vi "02 HEWH MINI Heat Up SM1.vi"(0 "Equipment":T6={"COM Port"="COM3", "MW100"="MW100", "AG34970"="A-34972A", "Chamber"="WT500"}, 2 "Semiphore":T3, 5 "Degree Setting":dbl=58.0, 7 "Flow rate setting":dbl=3.0, 11 "Error In":errorcluster) -> (15 "Error Out":errorcluster)   [LabVIEW 2009]
uses:
  EquipReferences.ctl
  HEWH Tank Indicator.ctl
  PowerElements.ctl
  TestedFlowratesScenarios.ctl
  <vilib>/Platform/fileVersionInfo.llb/FileVersionInformation.ctl
  ValveBankPositions.ctl
  Intellifaucet/Intellfaucet Mode.ctl
  <vilib>/Utility/file.llb/Write To Spreadsheet File (string).vi
  <vilib>/Analysis/NI_AALBase.lvlib
panel:
  in  "Expansion Tank?":bool
  out "FileVersionInfo Out":T1
  in  "Test Condition":T2=enum."Global, Tank"
  out "Chanel List":string
  out "Label Array":string[](array[string])
  out "Use Agilent?":bool
  out "Voltage":dbl=240.0
  out "T4":i32=10000
  out "COM Port":refnum<visa-resource-name>
  out "Serial Data In":string
  out "Error Serial":errorcluster
  in  "StopSerial":bool
  out "LAN IP Address":string="192.168.25.3"
  out "Computer Name":string
  out "Ver.":string
  out "MINI-HEATUP TEST STATUS":string
  in  "Stop":bool
  in  "Help":bool
  out "POWER":T4
  out "Tank Display":T5 {"TC6" format="%.2g"; "TIN" format="%.2g"; "TOUT" format="%.2g"; "Mean" format="%.2f"; "Std Dev" format="%.2f"; "TC5" format="%.2g"; "TC4" format="%.2g"; "TC3" format="%.2g"; "TC2" format="%.2g"; "TC1" format="%.2g"}
  in  "Function Tab":enum32{"Setup", "Test Status", "Charts"}(tab)
  out "MW100":refnum<visa-resource-name>
  out "FileName":path
  in  "Working File Directory":path=path "c:/data"
  out "T1":u32=250
  out "T2":u32=500
  out "T3":u32=500
  in  "Stability Sample Delay(s)":u32=30
  in  "Cold Water Available?":bool=TRUE
  in  "Save File Directory":path=path "c:/data"
  out "Init Complete":bool
  in  "Gallon Limit":dbl=40.0
  in  "Mean Tank Min":dbl=75.0
  in  "Min Tout":dbl=100.0
  in  "GEA2 HyperData":bool
  out "Data Array":string[][](array[string])
  in  "Status Tab":T7(tab)
  out "Flowrate adj":dbl=3.0
  out "Error Out 1":errorcluster
  out "Downspout Flow Chart":dbl(graph)=3.8899999999999997
  out "Temp Band(+/- F)":dbl=50.0
  out "Temp adj":dbl=3.0
  out "Error 5":errorcluster
  out "Downspout Flow Chart":dbl(graph)=3.8899999999999997
  out "Downspout Flow":dbl=3.8899999999999997
  out "Total Flow Out":dbl
  out "5.Top Source Indicator":bool
  in  "Flow Adjust Time (3s)":dbl=1.5
  in  "K(0.1)":dbl=0.1
  out "Gallon Limit 2":dbl=40.0
  out "Mean Tank Min 2":dbl
  out "Min Tout 2":dbl
  out "Heat Source Indicator":bool
  in  "SkipStabilize":bool
  out "error stabilize":errorcluster
  out "Elapsed Time (secs)":dbl format="%.2f"
  out "LoggingStopped":bool=TRUE
  out "Error History":string[](array[string])
  out "Com History":string[](array[string])
  out "error datalogging":errorcluster={"status"=TRUE, "code"=-1073807346, "source"="VISA Read in Gather Test Data.vi"}
  out "St.Logging":bool
  out "Number of Records":i32
  out "Test Data":string[][](array[string])
  in  "Graph Tab":enum32{"Temperature", "Power", "Gallons"}(tab)
  out "Temps":T8(graph) caption="Waveform Chart"
  out "Ave Temp":dbl format="%0.2f"
  out "Watt Chart":T9(graph)
  out "Watts":dbl
  out "Gallons Chart":dbl(graph)
  out "Gallons":dbl
  out "Elapsed Time":dbl format="%<%H:%M:%S>t"
  in  "Stop Logging":bool
  out "Local?":bool
  # "Draw Until:"
  # "Total Gallons Drawn >"
  # "OR"
  # "Mean Temp >="
  # "OR"
  # "Tout <="
  # "\"1.\tAfter unit has been stable for 30+/-5 minutes, Open valve,\n and draw 10.75 +/- .25 gallons of water at a rate of 3+/-.25 gpm.\""
  # "First, Allow the water temp and flow to stabilize in the downspout,\nthen switch to the tank."
  # "\"5.\tOpen valve and draw water at 3+/-.25 gpm until the Upper Element \nenergizes.  Water draw must stop within 5 seconds after Upper Element \nenergizes.  NOTE: when running the unit in e-Heat mode, (no upper \nelement) draw 40+/-0.25 gallons of water.\""
  # "Wait for stabilization.  Checks heat sources every second.  \nIf the heat sources are both off, the water heater is stabilized. \nFor StdElect. Looks at the heating element.  For other heating\nmodes, looks at the RS232 feedback on fans and compressor."
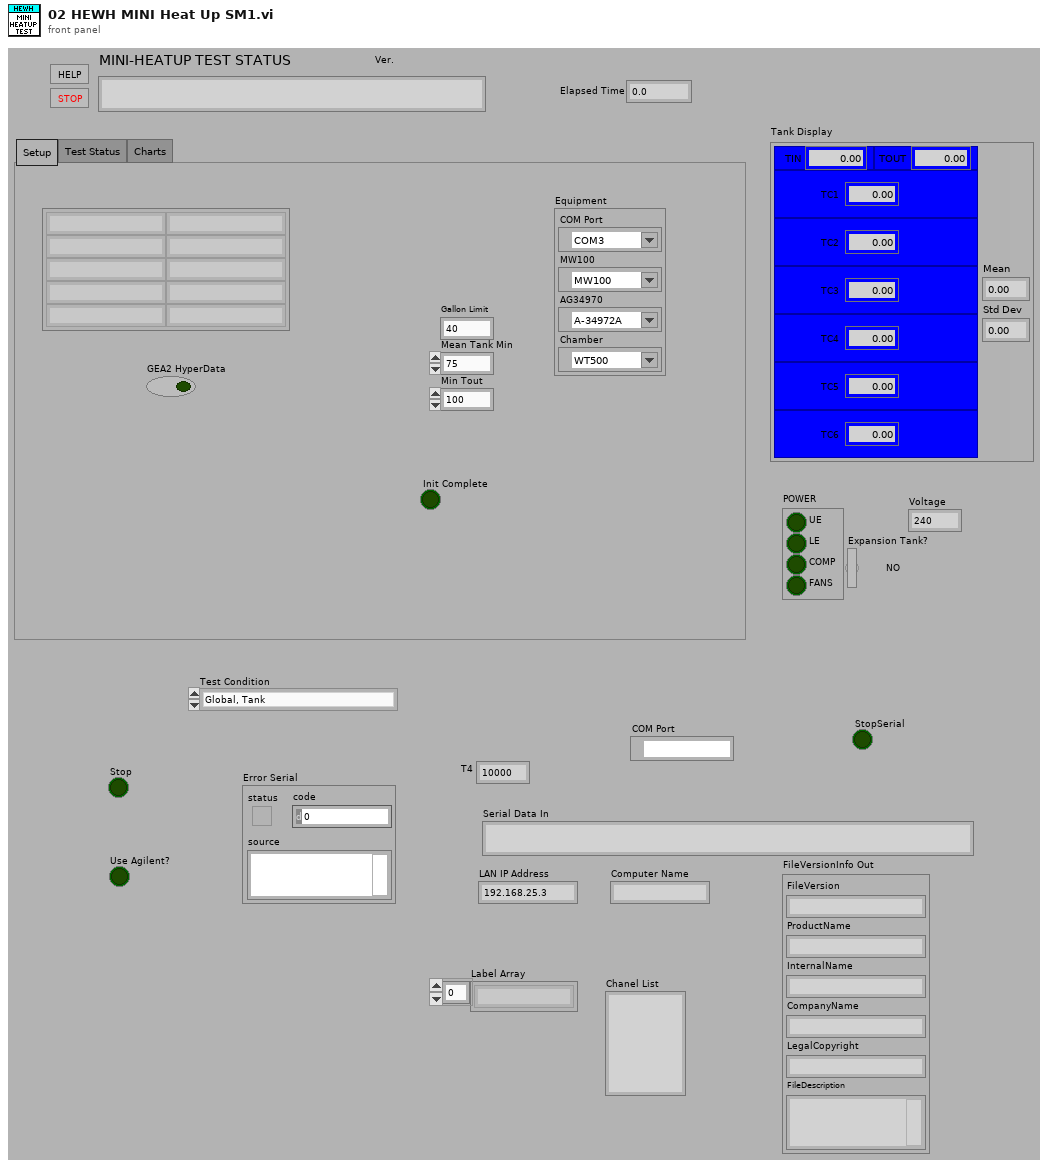
[diagram p1: front panel]
types:
  T1 = typedef "FileVersionInformation.ctl" = cluster{"FileVersion":string, "ProductName":string, "InternalName":string, "CompanyName":string, "LegalCopyright":string, "FileDescription":string}
  T2 = typedef "TestedFlowratesScenarios.ctl" = enum16{"DRK500,Station1", "DRK375,Lab", "SRK500,Station1,5GPM FR", "DRK375,STATION3,1/2\"HOSE", "DRK500,Station1,downspout", "DRK375,Station3,thruEcocute", "DRK375,Station3,purge", "Build2,2B,Purge", "Global, Purge", "Global, Tank"}
  T3 = typedef "Semaphore RefNum" = refnum<k1>
  T4 = typedef "PowerElements.ctl" = cluster{"UE":bool, "LE":bool, "COMP":bool, "FANS":bool}
  T5 = typedef "HEWH Tank Indicator.ctl" = cluster{"TC1-D":bool, "TC2-D":bool, "TC3-D":bool, "TC4-D":bool, "TC5-D":bool, "RTD_IN":bool, "RTDOUT":bool, "TC1":dbl, "TC2":dbl, "TC3":dbl, "TC4":dbl, "TC5":dbl, "TIN":dbl, "TOUT":dbl, "Std Dev":dbl, "Mean":dbl, "TC6-D":bool, "TC6":dbl}
  T6 = typedef "EquipReferences.ctl" = cluster{"COM Port":refnum<visa-resource-name>, "MW100":refnum<visa-resource-name>, "AG34970":refnum<visa-resource-name>, "Chamber":refnum<visa-resource-name>}
  T7 = enum32{"Program Controls", "Feedback 4", "External Program Controls 2", "Feedback 10"}
  T8 = cluster{"Tc Tree[0]":dbl, "Tc Tree[1]":dbl, "Tc Tree[2]":dbl, "Tc Tree[3]":dbl, "Tc Tree[4]":dbl, "Tc Tree[5]":dbl}[]
  T9 = cluster{"[0]":dbl, "[1]":dbl, "[2]":dbl, "[3]":dbl, "[4]":dbl, "[5]":dbl}[]
  T10 = typedef "Intellfaucet Mode.ctl" = enum16{"Adjust Temp", "Adjust Flow", "Start Flow", "Stop Flow"}
  T11 = typedef "ValveBankPositions.ctl" = enum16{"Heating", "Purge", "Resting", "Draw"}
  T12 = enum16{"Computation Start", "Computation stop", "Reset Computation", "Clear Computation"}[]
  T13 = typedef "PowerData.ctl" = cluster{"Voltage":dbl, "Current":dbl, "Power":dbl, "WattHours":dbl}
  T14 = cluster{"Tc Tree[0]":dbl, "Tc Tree[1]":dbl, "Tc Tree[2]":dbl, "Tc Tree[3]":dbl, "Tc Tree[4]":dbl, "Tc Tree[5]":dbl}
  T15 = cluster{"[0]":dbl, "[1]":dbl, "[2]":dbl, "[3]":dbl, "[4]":dbl, "[5]":dbl}
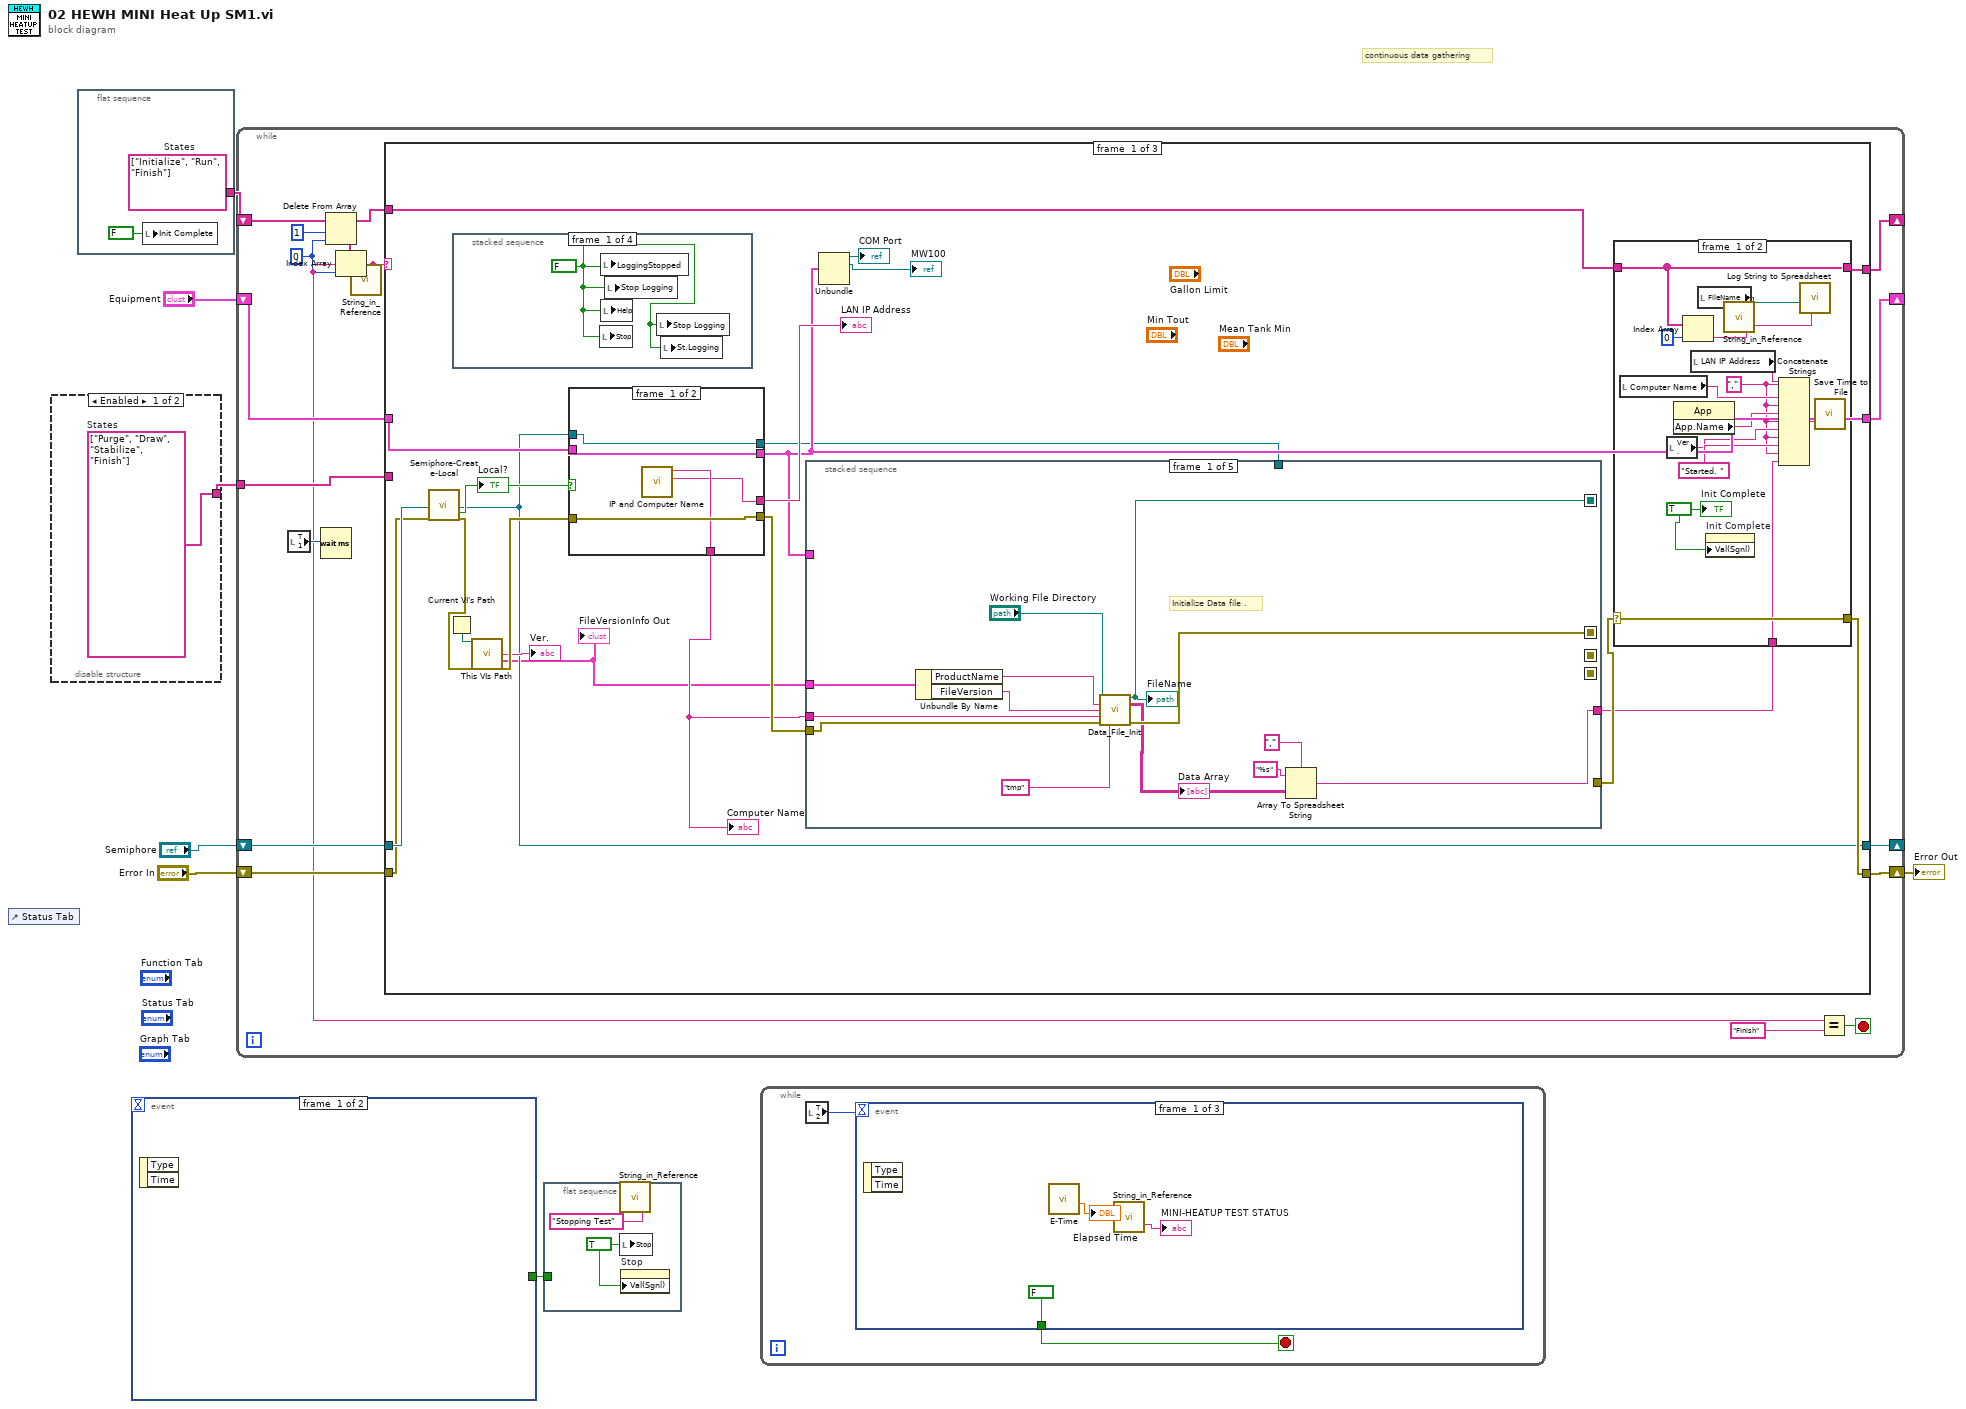
[diagram p0: block diagram]
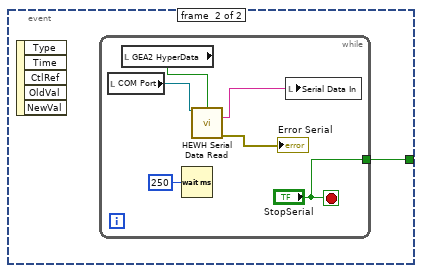
[diagram p2: hidden frame]
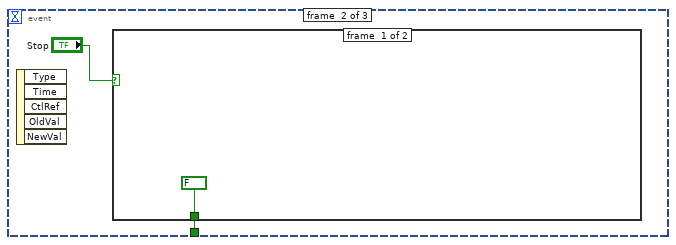
[diagram p3: hidden frame]
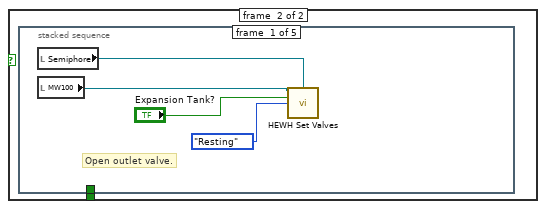
[diagram p4: hidden frame]
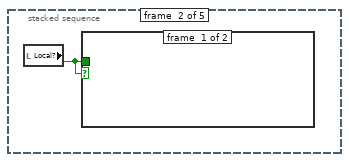
[diagram p5: hidden frame]
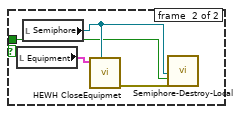
[diagram p6: hidden frame]
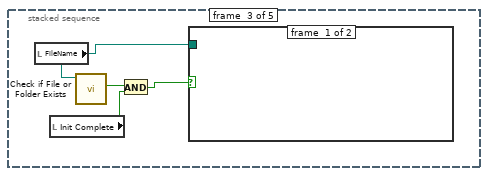
[diagram p7: hidden frame]
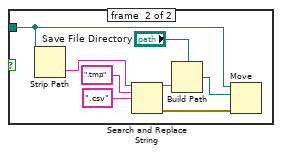
[diagram p8: hidden frame]
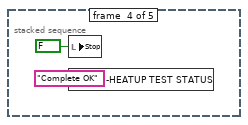
[diagram p9: hidden frame]
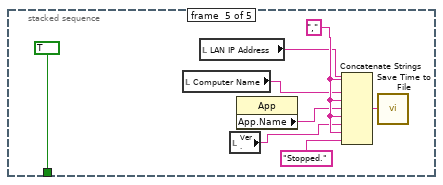
[diagram p10: hidden frame]
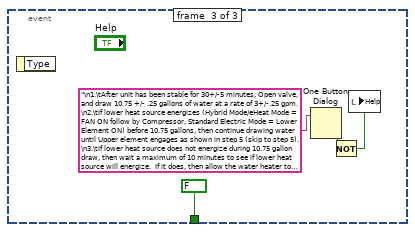
[diagram p11: hidden frame]
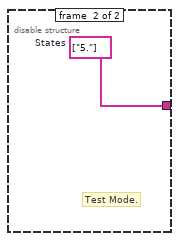
[diagram p12: hidden frame]
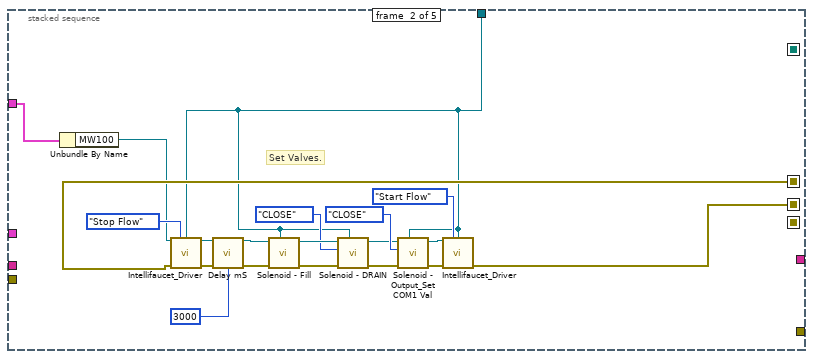
[diagram p13: hidden frame]
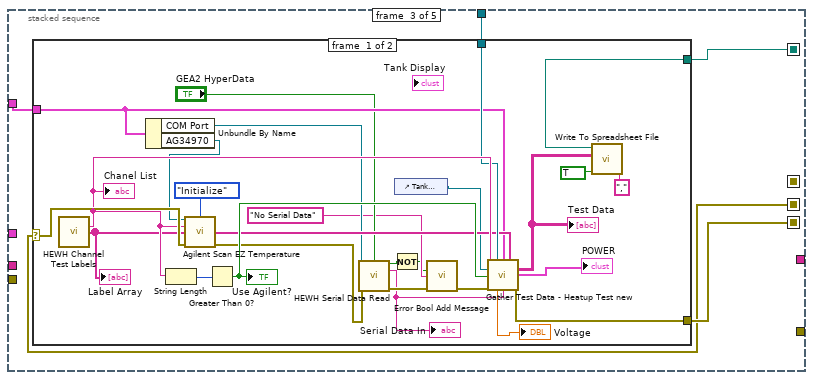
[diagram p14: hidden frame]
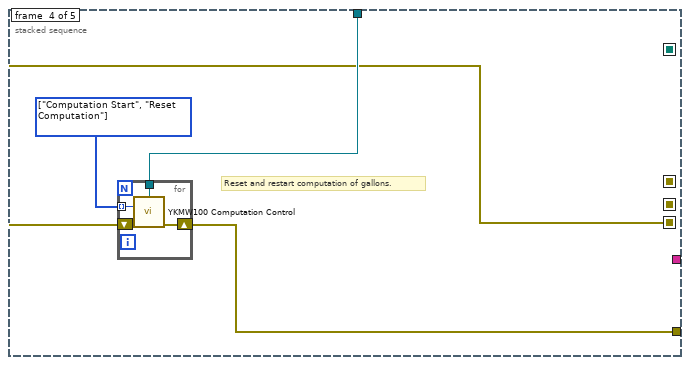
[diagram p16: hidden frame]
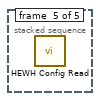
[diagram p17: hidden frame]
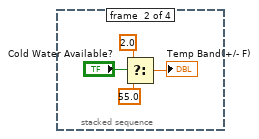
[diagram p18: hidden frame]
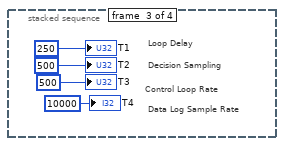
[diagram p19: hidden frame]
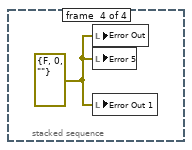
[diagram p20: hidden frame]
diagram:
  # "continuous data gathering"
  n1 = control-ref of="Status Tab"() -> ()  [unwired: 1 out]
  n2 = disable-structure shown="Enabled" {
    disable-tunnel: [w8 w9] -> w5
    frame #0 {
      w8 = string[] ["Purge", "Draw", "Stabilize", "Finish"]  # States
    }
    frame #1 {
      w9 = string[] ["5."]  # States
      # "Test Mode."
    }
  }
  n3 = flat-sequence {
    tunnel: [w11] -> w7
    frame #0 {
      w11 = string[] ["Initialize", "Run", "Finish"]  # States
      n4 = local write "Init Complete"(FALSE ("Init Complete")) -> ()
    }
  }
  n5 = event shown="[1] \"Init Complete\", \"Stop Logging\": Value Change" {
    selector: _ -> [_ _]
    dyn-events: _ -> [_ _]
    timeout: _ -> [_ _]
    tunnel: [_ w12] -> w1
    event #0 {
      n6 = event-data() -> ()  [unwired: 1 in, 2 out]
    }
    event #1 {
      n7 = event-data() -> ()  [unwired: 1 in, 5 out]
      n8 = while {
        tunnel: ["StopSerial"] -> w12
        stop <- "StopSerial" stop-if-true
        n9 = local read "COM Port"() -> (w15:refnum<visa-resource-name>)
        n10 = local read "GEA2 HyperData"() -> (w13:bool)
        n11 = Wait (ms)(milliseconds to wait=u32 250) -> ()  [unwired: 1 out]
        n12 = call "HEWH Serial Data Read.vi"("Serial Port Ref"=w15, "GEA2 HyperData"=w13) -> ("Read String"=w17:string, "error out"=→"Error Serial":errorcluster)  [unwired: 11 in, 1 out]
        n13 = local write "Serial Data In"(w17) -> ()
      }
    }
  }
  n14 = while {
    shift-right: [w31] -> _
    shift-left: w7 -> [w35]
    shift-right: [w29] -> w6
    shift-left: "Error In" -> [w28]
    shift-right: [w25] -> _
    shift-left: "Equipment" -> [w21]
    tunnel: w5 -> [w24]
    shift-right: [w22] -> _
    shift-left: "Semiphore" -> [w23]
    stop <- w27 stop-if-true
    w32 = 0 ("index")
    n15 = local read "T1"() -> (w20:u32)
    n16 = Wait (ms)(milliseconds to wait=w20) -> ()  [unwired: 1 out]
    n17 = Delete From Array(array=w35, length=1, index=w32) -> (deleted portion=w33:string[], array with subset deleted=w30:string[])
    n18 = Index Array(array=w33, index=w32) -> (element=w19:string)
    n19 = call "String_in_Reference.vi"("String"=w19) -> ()  [unwired: 18 in, 1 out]
    n20 = case shown="\"Run\"" w19 {
      tunnel: [w54 w170 w474] -> w31
      tunnel: w30 -> [w55 w170 w475]
      tunnel: [w56 w173 w476] -> w29
      tunnel: w28 -> [w51 w174 w472]
      tunnel: w21 -> [w57 w172 w471]
      tunnel: [w40 w172 w471] -> w25
      tunnel: w24 -> [_ w175 _]
      tunnel: w23 -> [w52 w171 w473]
      tunnel: [w45 w171 w473] -> w22
      frame #0 {
        n21 = call "Semiphore-Create-Local.vi"("Semiphore"=w52, "error in (no error)"=w51) -> ("semaphore"=w45:T3, "Local?"=w53:bool, "error out"=w49:errorcluster)  [unwired: 15 in]
        "Local?" <- w53
        n22 = Current VI's Path() -> (path=w50:path)
        n23 = stacked-sequence {
          frame #0 {
            w130 = FALSE ("BottomHeater")
            n24 = local write "Stop"(w130) -> ()
            n25 = local write "LoggingStopped"(w130) -> ()
            n26 = local write "Help"(w130) -> ()
            n27 = local write "Stop Logging"(w130) -> ()
            n28 = local write "Stop Logging"(w130) -> ()
            n29 = local write "St.Logging"(w130) -> ()
          }
          frame #1 {
            n30 = Select(t=2.0, s="Cold Water Available?", f=55.0) -> (s? t:f=→"Temp Band(+/- F)":dbl)
          }
          frame #2 {
            # "Data Log Sample Rate"
            # "Loop Delay"
            # "Decision Sampling"
            # "Control Loop Rate"
            "T1" <- u32 250
            "T2" <- u32 500 ("T2")
            "T3" <- u32 500 ("T3")
            "T4" <- 10000 ("T4")
          }
          frame #3 {
            w139 = errorcluster {"status"=FALSE, "code"=0, "source"=""} ("Error Out")
            n31 = local write "Error Out"(w139) -> ()
            n32 = local write "Error 5"(w139) -> ()
            n33 = local write "Error Out 1"(w139) -> ()
          }
        }
        n34 = call "This VIs Path.vi"("path"=w50, "error in (no error)"=w49) -> ("File Version Info"=→"Ver.":string, "FileVersionInfo Out"=w36:T1, "error out"=w48:errorcluster)  [unwired: 9 in, 2 out]
        "FileVersionInfo Out" <- w36
        n35 = case shown="False" w53 {
          tunnel: w48 -> [w161 w168]
          tunnel: w57 -> [w160 w165]
          tunnel: [w160 w166] -> w40
          tunnel: [w161 w167] -> w41
          tunnel: w45 -> [w157 w162]
          tunnel: [w159 w164] -> w38
          tunnel: [w158 w163] -> w44
          tunnel: [w157 w162] -> w39
          frame #0 {
            n36 = call "IP and Computer Name.vi"() -> ("IP Address"=w158:string, "Computer Name"=w159:string)  [unwired: 10 in]
          }
          frame #1 {
            n37 = local write "Semiphore"(w162) -> ()
            n38 = call "HEWH InitializeEquipmet.vi"("Semiphore"=w162, "Error In"=w168, "Equipment"=w165) -> ("Error Out"=w167:errorcluster, "Computer Name"=w164:string, "LAN IP Address"=w163:string, "Equipment Out"=w166:T6)  [unwired: 5 in]
            n39 = local write "Equipment"(w166) -> ()
          }
        }
        "Computer Name" <- w38
        "LAN IP Address" <- w44
        n40 = stacked-sequence {
          seq-local: [_ w76 _ _ _] -> [_ _ w90 _ _]
          seq-local: [w68 _ _ _ _] -> [_ w75 _ _ _]
          seq-local: [_ _ w92 _ _] -> [_ _ _ w122 _]
          seq-local: [w66 _ _ _ _] -> [_ _ w91 _ _]
          tunnel: [_ _ _ w124 _] -> w42
          tunnel: w38 -> [w70 _ _ _ _]
          tunnel: w41 -> [w69 _ _ _ _]
          tunnel: w40 -> [_ w72 w94 _ _]
          tunnel: w39 -> [_ w73 w93 w123 _]
          tunnel: [w62 _ _ _ _] -> w37
          tunnel: w36 -> [w60 _ _ _ _]
          frame #0 {
            # "Initialize Data file ."
            n41 = Unbundle By Name(w60) -> ("ProductName"=w59:string, "FileVersion"=w58:string)
            n42 = call "Data_File_Init.vi"("Data File Directory"="Working File Directory", "Test_Type In:"=w59, "Version In:"=w58, "Computer Name In:"=w70, "error in (no error)"=w69, "File Extension:"="tmp") -> ("FileName"=w66:path, "Data Array"=w63:string[][], "error out"=w68:errorcluster)  [unwired: 7 in]
            "FileName" <- w66
            "Data Array" <- w63
            n43 = Array To Spreadsheet String(delimiter (Tab)=",", array=w63, 3:"%s" ("format string")) -> (spreadsheet string=w62:string)
          }
          frame #1 {
            # "Set Valves."
            n44 = Unbundle By Name(w72) -> ("MW100"=w71:refnum<visa-resource-name>)
            n45 = call "Intellifaucet_Driver.vi"("VISA session"=w71, "Mode"=Intellfaucet_Mode."Stop Flow", "Semiphore"=w73, "Error In"=w75) -> ("VISA session out"=w85:refnum<visa-resource-name>, "Error Out"=w79:errorcluster)  [unwired: 10 in]
            n46 = call "Delay mS.vi"("Error In"=w79, "milliseconds to wait"=u32 3000) -> ("Error Out"=w81:errorcluster)  [unwired: 13 in]
            n47 = call "Solenoid - Fill.vi"("Semiphore"=w73, "Error In"=w81, "VISA session"=w85) -> ("Error Out"=w80:errorcluster, "dup VISA session"=w82:refnum<visa-resource-name>)  [unwired: 7 in]
            n48 = call "Solenoid - DRAIN.vi"("Semiphore"=w73, "Error In"=w80, "VALVE OPEN CLOSE"=enum8{"OPEN", "CLOSE"}."CLOSE", "VISA session"=w82) -> ("Error Out"=w84:errorcluster, "dup VISA session"=w83:refnum<visa-resource-name>)  [unwired: 6 in]
            n49 = call "Solenoid - Output_Set COM1 Val.vi"("Semiphore"=w73, "Error In"=w84, "OPEN CLOSE"=enum8{"CLOSE", "OPEN"}."CLOSE", "VISA session"=w83) -> ("Error Out"=w78:errorcluster, "dup VISA session"=w74:refnum<visa-resource-name>)  [unwired: 6 in]
            n50 = call "Intellifaucet_Driver.vi"("VISA session"=w74, "Mode"=Intellfaucet_Mode."Start Flow", "Semiphore"=w73, "Error In"=w78) -> ("Error Out"=w76:errorcluster)  [unwired: 10 in, 1 out]
          }
          frame #2 {
            n51 = case shown="No Error" w90 {
              selector: w90 -> [w120 w121]
              tunnel: w94 -> [w110 _]
              tunnel: w93 -> [w114 _]
              tunnel: [w107 w121] -> w92
              tunnel: w91 -> [w104 _]
              frame #0 {
                n52 = call "HEWH Channel Test Labels.vi"() -> ("Chanel List"=w115:string, "Label List"=w112:string[])  [unwired: 13 in, 1 out]
                "Chanel List" <- w115
                "Label Array" <- w112
                n53 = Unbundle By Name(w110) -> ("COM Port"=w109:refnum<visa-resource-name>, "AG34970"=w108:refnum<visa-resource-name>)
                n54 = String Length(string=w115) -> (length=w118:i32)
                n55 = call "Agilent Scan EZ Temperature.vi"("VISA Resource Name"=w108, "Control"=enum16{"Initialize", "Read", "Experiment"}."Initialize", "Channel Input"=w115, "error in (no error)"=w120) -> ("error out"=w111:errorcluster)  [unwired: 8 in, 3 out]
                n56 = Greater Than 0?(x=w118) -> (x > 0?=w116:bool)
                "Use Agilent?" <- w116
                n57 = call "HEWH Serial Data Read.vi"("Serial Port Ref"=w109, "GEA2 HyperData"="GEA2 HyperData", "error in (no error)"=w111) -> ("Serial Read OK"=w97:bool, "Read String"=w103:string, "error out"=w117:errorcluster)  [unwired: 10 in]
                "Serial Data In" <- w103
                n58 = Not(x=w97) -> (.not. x?=w95:bool)
                n59 = control-ref of="Tank Display"() -> (w102:refnum<vi>)
                n60 = call "Error Bool Add Message.vi"("Error?"=w95, "Message"="No Serial Data", "Error In"=w117) -> ("Error Out"=w98:errorcluster)  [unwired: 12 in]
                n61 = call "Gather Test Data - Heatup Test new.vi"("Agilent Scan List"=w115, "Semiphore"=w114, "Equipment"=w110, "Tank Display Ref"=w102, "Agilent?"=w116, "error in (no error)"=w98, "Serial Data In"=w103, "Agilent Label Array"=w112) -> ("Output Data"=w101:string[][], "POWER"=→"POWER":T4, "Voltage"=→"Voltage":dbl, "error out"=w107:errorcluster)  [unwired: 2 in, 2 out]
                "Test Data" <- w101
                n62 = call-poly <vilib>:"Write To Spreadsheet File.vi"("delimiter (\\t)"="," ("delimiter (\\t)"), "append to file? (new file:F)"=TRUE, "2D data"=w101, "file path (dialog if empty)"=w104) -> ()  [unwired: 4 in, 1 out]
              }
              frame #1 {
              }
            }
          }
          frame #3 {
            w125 = T12 [enum."Computation Start", enum."Reset Computation"] items=["Computation Start", "Computation stop", "Reset Computation", "Clear Computation"]
            # "Reset and restart computation of gallons."
            n63 = for {
              tunnel: w125 -> [w127] mode=indexing
              shift-right: [w128] -> w124
              shift-left: w122 -> [w129]
              tunnel: w123 -> [w126]
              n64 = call "YKMW100 Computation Control.vi"("Semiphore"=w126, "Mode"=w127, "error in (no error)"=w129) -> ("error out"=w128:errorcluster)  [unwired: 11 in, 1 out]
            }
          }
          frame #4 {
            n65 = call "HEWH Config Read.vi"() -> ()  [unwired: 14 in, 2 out]
          }
        }
        n66 = Unbundle(w40) -> ("COM Port"=→"COM Port":refnum<visa-resource-name>, "MW100"=→"MW100":refnum<visa-resource-name>)  [unwired: 2 out]
        n67 = case shown="No Error" w42 {
          selector: w42 -> [w154 w156]
          tunnel: [w149 string[] ["Finish"] ("States")] -> w54
          tunnel: w55 -> [w149 _]
          tunnel: [w154 w156] -> w56
          tunnel: w37 -> [w140 _]
          frame #0 {
            w141 = ","
            w148 = TRUE ("Init Complete")
            n68 = local read "Computer Name"() -> (w142:string)
            n69 = local read "Ver."() -> (w143:string)
            n70 = property class="App"() -> ("App.Name"=w145:string)  [unwired: 2 in, 2 out]
            n71 = Index Array(array=w149, index=0) -> (element=w152:string)
            n72 = local read "LAN IP Address"() -> (w146:string)
            n73 = local read "FileName"() -> (w151:path)
            n74 = property on="Init Complete" class="Bool (strict)"("Val(Sgnl)"=w148) -> ()  [unwired: 2 in, 2 out]
            n75 = call "String_in_Reference.vi"("String"=w152) -> ("String Out"=w150:string)  [unwired: 18 in]
            n76 = Concatenate Strings(w146, w141, w142, w141, w145, w141, w143, w141, "Started. " ("string"), w141, w140) -> (w147:string)
            n77 = call "Log String to Spreadsheet.vi"("String"=w150, "FileName"=w151) -> ()  [unwired: 9 in, 1 out]
            n78 = call "Save Time to File.vi"("String"=w147) -> ()  [unwired: 13 in, 2 out]
            "Init Complete" <- w148
          }
          frame #1 {
            n79 = call <vilib>:"Simple Error Handler.vi"("error in (no error)"=w156) -> ()  [unwired: 4 in, 5 out]
          }
        }
      }
      frame #1 {
        n80 = while {
          shift-right: [w189] -> _
          shift-left: w175 -> [w191]
          tunnel: w174 -> [w184]
          tunnel: [w190] -> w173
          tunnel: w172 -> [w186]
          tunnel: w171 -> [w185]
          stop <- w180 stop-if-true
          w192 = 0 ("index")
          # "Water Draw Test Sequence"
          n81 = local read "Stop Logging"() -> (w177:bool)
          n82 = Delete From Array(array=w191, length=1, index=w192) -> (deleted portion=w193:string[], array with subset deleted=w188:string[])
          n83 = Index Array(array=w193, index=w192) -> (element=w179:string)
          n84 = flat-sequence {
            tunnel: w184 -> [w199]
            tunnel: [w199] -> w183
            tunnel: [w195] -> w181
            tunnel: w176 -> [w195]
            frame #0 {
              n85 = local read "FileName"() -> (w198:path)
              n86 = control-ref of="Status Tab"() -> (w196:refnum<vi>)
              n87 = call "Tab Control - Change to TabName MiniHeatup.vi"("Label.Text"=w195, "Status Tab 3"=w196) -> ()  [unwired: 9 in]
              n88 = call "String_in_Reference.vi"("String"=w195) -> ("String Out"=w197:string)  [unwired: 18 in]
              n89 = call "Log String to Spreadsheet.vi"("String"=w197, "FileName"=w198) -> ()  [unwired: 9 in, 1 out]
            }
          }
          n90 = local read "T1"() -> (w182:u32)
          n91 = Wait (ms)(milliseconds to wait=w182) -> ()  [unwired: 1 out]
          n92 = Select(t="Finish", s=w177, f=w179) -> (s? t:f=w176:string)
          n93 = case shown="\"Draw\"" w176 {
            tunnel: w183 -> [w201 w261 w297 w391]
            tunnel: [w207 w276 w310 w387] -> w190
            tunnel: [w206 w275 w311 w395] -> w189
            tunnel: w188 -> [w205 w274 w312 w395]
            tunnel: w186 -> [w204 w256 _ _]
            tunnel: w185 -> [w202 w255 w302 w390]
            frame #0 {
              n94 = while {
                tunnel: w204 -> [_]
                tunnel: w201 -> [w213]
                tunnel: [w236] -> w203
                tunnel: w202 -> [w225]
                shift-right: [w216] -> _
                shift-left: FALSE -> [w215]
                i -> [w221]
                stop <- w219 stop-if-true
                n95 = flat-sequence {
                  tunnel: [w237] -> w214
                  tunnel: w213 -> [w237]
                  frame #0 {
                    n96 = local read "T2"() -> (w238:u32)
                    n97 = Wait (ms)(milliseconds to wait=w238) -> ()  [unwired: 1 out]
                  }
                }
                n98 = local read "Use Agilent?"() -> (w209:bool)
                n99 = local read "Chanel List"() -> (w228:string)
                n100 = local read "Equipment"() -> (w229:T6)
                n101 = local read "Serial Data In"() -> (w211:string)
                n102 = control-ref of="Tank Display"() -> (w227:refnum<vi>)
                n103 = local read "Label Array"() -> (w210:string[])
                n104 = call "Gather Test Data - Heatup Test new.vi"("Agilent Scan List"=w228, "Semiphore"=w225, "Equipment"=w229, "Tank Display Ref"=w227, "Agilent?"=w209, "error in (no error)"=w214, "Serial Data In"=w211, "Agilent Label Array"=w210) -> ("Output Data"=w223:string[][], "POWER"=w226:T4, "Voltage"=w208:dbl, "error out"=w224:errorcluster)  [unwired: 2 in, 2 out]
                n105 = Equal To 0?(x=w221) -> (x = 0?=w220:bool)
                n106 = local read "St.Logging"() -> (w212:bool)
                n107 = local write "Voltage"(w208) -> ()
                n108 = local write "Test Data"(w223) -> ()
                n109 = local write "POWER"(w226) -> ()
                n110 = Unbundle(w226) -> ("UE"=w231:bool, "LE"=w232:bool, "COMP"=w233:bool, "FANS"=w218:bool)
                n111 = Compound Arithmetic op=AND(invert w231, invert w232, invert w233, invert w218) -> (w216:bool)
                n112 = Not(x=w216) -> (.not. x?=→"Heat Source Indicator":bool)
                n113 = And(x=w215, y=w216) -> (x .and. y?=w217:bool)
                n114 = Compound Arithmetic op=OR(w217, "SkipStabilize", w212) -> (w219:bool)
                n115 = Compound Arithmetic op=OR(w220, w219) -> (w222:bool)
                n116 = case shown="True" w222 {
                  tunnel: w223 -> [_ w241]
                  frame #0 {
                  }
                  frame #1 {
                    n117 = local read "FileName"() -> (w244:path)
                    n118 = Index Array(array=w241, index (row)=1) -> (element=w240:string[])  [unwired: 1 in]
                    n119 = call-poly <vilib>:"Write To Spreadsheet File.vi"("delimiter (\\t)"="," ("delimiter (\\t)"), "append to file? (new file:F)"=TRUE, "1D data"=w240, "file path (dialog if empty)"=w244) -> ()  [unwired: 4 in, 1 out]
                  }
                }
                n120 = case shown="True" w216 {
                  frame #0 {
                  }
                  frame #1 {
                    n121 = Wait (ms)(milliseconds to wait="Stability Sample Delay(s)") -> ()  [unwired: 1 out]
                  }
                }
                n122 = call "E-Time.vi"("error in (no error)"=w224) -> ("error out"=w236:errorcluster, "Elapsed Time (sec)"=→"Elapsed Time (secs)":dbl)  [unwired: 8 in, 1 out]
              }
              n123 = case shown="Error" w203 {
                selector: w203 -> [w246 w248]
                tunnel: [w247 string[] ["Finish"] ("States")] -> w206
                tunnel: w205 -> [w247 _]
                tunnel: [w246 w248] -> w207
                frame #0 {
                }
                frame #1 {
                  n124 = Unbundle By Name(w248) -> ("source"=w253:string)
                  n125 = local read "FileName"() -> (w250:path)
                  n126 = Concatenate Strings("Error: " ("string"), w253) -> (w251:string)
                  n127 = call "String_in_Reference.vi"("String"=w251) -> ("String Out"=w249:string)  [unwired: 18 in]
                  n128 = call "Log String to Spreadsheet.vi"("String"=w249, "FileName"=w250) -> ()  [unwired: 9 in, 1 out]
                  "error stabilize" <- w248
                }
              }
            }
            frame #1 {
              n129 = Unbundle By Name(w256) -> ("MW100"=w257:refnum<visa-resource-name>)
              n130 = call "HEWH Totalize Flow Control.vi"("VISA session"=w257, "Semiphore"=w255, "Totalize Flow"=FALSE, "error in (no error)"=w261) -> ("error out"=w259:errorcluster)  [unwired: 10 in, 1 out]
              n131 = local read "FileName"() -> (w265:path)
              n132 = control-ref of="Downspout Flow Chart"() -> (w270:refnum<vi>)
              n133 = local read "Test Condition"() -> (w263:T2)
              n134 = local read "Temp Band(+/- F)"() -> (w269:dbl)
              n135 = flat-sequence {
                tunnel: "PurgeBegins" ("string") -> [w284]
                tunnel: w259 -> [w283]
                tunnel: [w282] -> w267
                tunnel: w265 -> [w281]
                frame #0 {
                  n136 = call "String_in_Reference.vi"("String"=w284) -> ()  [unwired: 18 in, 1 out]
                  n137 = call "Log String to Spreadsheet.vi"("String"=w284, "error in (no error)"=w283, "FileName"=w281) -> ("error out"=w282:errorcluster)  [unwired: 8 in]
                }
              }
              n138 = call "Purge Water Sequence SM.vi"("Degree Setting"="Degree Setting", "Equipment"=w256, "Semiphore"=w255, "Flow rate setting"="Flow rate setting", "Temp Band(+/- F)"=w269, "Error In"=w267, "Flow Chart Ref"=w270, "Test Condition"=w263) -> ("Flow rate setting out"=→"Flowrate adj":dbl, "Temp Setting Out"=→"Temp adj":dbl, "Error Out"=w266:errorcluster)  [unwired: 2 in, 3 out]
              n139 = flat-sequence {
                tunnel: w266 -> [w280]
                tunnel: [w279] -> w260
                tunnel: w265 -> [w278]
                tunnel: "PurgeEnds" ("string") -> [w277]
                frame #0 {
                  n140 = call "String_in_Reference.vi"("String"=w277) -> ()  [unwired: 18 in, 1 out]
                  n141 = call "Log String to Spreadsheet.vi"("String"=w277, "error in (no error)"=w280, "FileName"=w278) -> ("error out"=w279:errorcluster)  [unwired: 8 in]
                }
              }
              n142 = case shown="Error" w260 {
                selector: w260 -> [w285 w287]
                tunnel: [w286 string[] ["Finish"] ("States")] -> w275
                tunnel: w274 -> [w286 _]
                tunnel: [w285 w287] -> w276
                frame #0 {
                }
                frame #1 {
                  n143 = Unbundle By Name(w287) -> ("source"=w292:string)
                  n144 = local read "FileName"() -> (w289:path)
                  n145 = Concatenate Strings("Error: " ("string"), w292) -> (w290:string)
                  n146 = call "String_in_Reference.vi"("String"=w290) -> ("String Out"=w288:string)  [unwired: 18 in]
                  n147 = call "Log String to Spreadsheet.vi"("String"=w288, "FileName"=w289) -> ()  [unwired: 9 in, 1 out]
                  "Error Out 1" <- w287
                }
              }
            }
            frame #2 {
              n148 = local read "Expansion Tank?"() -> (w295:bool)
              n149 = local read "MW100"() -> (w296:refnum<visa-resource-name>)
              n150 = local read "Flowrate adj"() -> (w307:dbl)
              n151 = local read "Temp adj"() -> (w299:dbl)
              n152 = call "HEWH Set Valves.vi"("VISA session"=w296, "Semiphore"=w302, "Expansion Tank?"=w295, "Valve Bank Setting"=ValveBankPositions."Draw", "Error In"=w297) -> ("dup VISA session"=w303:refnum<visa-resource-name>, "Error Out"=w304:errorcluster)  [unwired: 9 in]
              n153 = call "HEWH Totalize Flow Control.vi"("VISA session"=w303, "Semiphore"=w302, "Totalize Flow"=TRUE, "error in (no error)"=w304) -> ("error out"=w306:errorcluster)  [unwired: 10 in, 1 out]
              n154 = while {
                shift-right: [w349] -> w309
                shift-left: w306 -> [w357]
                shift-right: [w368] -> w301
                shift-left: w307 -> [w369]
                tunnel: w302 -> [w340]
                tunnel: [w340] -> w308
                tunnel: [w366] -> w305
                shift-right: [w339] -> w300
                shift-left: w299 -> [w336]
                i -> [w353]
                stop <- w351 stop-if-true
                n155 = local read "Serial Data In"() -> (w332:string)
                n156 = local read "Use Agilent?"() -> (w330:bool)
                n157 = local read "Label Array"() -> (w331:string[])
                n158 = local read "T3"() -> (w365:u32)
                n159 = local read "Flow rate setting"() -> (w342:dbl)
                n160 = local read "Chanel List"() -> (w361:string)
                n161 = local read "Degree Setting"() -> (w343:dbl)
                n162 = Wait (ms)(milliseconds to wait=w365) -> ()  [unwired: 1 out]
                n163 = local read "Equipment"() -> (w362:T6)
                n164 = control-ref of="Tank Display"() -> (w360:refnum<vi>)
                n165 = call "Gather Test Data - Heatup Test new.vi"("Agilent Scan List"=w361, "Semiphore"=w340, "Equipment"=w362, "Tank Display Ref"=w360, "Agilent?"=w330, "error in (no error)"=w357, "Serial Data In"=w332, "Agilent Label Array"=w331) -> ("Output Data"=w345:string[][], "POWER"=w355:T4, "Voltage"=w333:dbl, "error out"=w356:errorcluster)  [unwired: 2 in, 2 out]
                n166 = local write "Voltage"(w333) -> ()
                n167 = local write "Test Data"(w345) -> ()
                n168 = local read "MW100"() -> (w354:refnum<visa-resource-name>)
                n169 = local write "POWER"(w355) -> ()
                n170 = call "E-Time.vi"("error in (no error)"=w356) -> ("error out"=w367:errorcluster, "Elapsed Time (sec)"=w347:dbl)  [unwired: 8 in, 1 out]
                n171 = call "Array_Search_For_Num.vi"("N Rows of Data"=w345, "Title?"="Tc_down") -> ("number"=w344:dbl)  [unwired: 12 in, 1 out]
                n172 = call "Array_Search_For_Num.vi"("N Rows of Data"=w345, "Title?"="FLOW(GPM)") -> ("number"=w358:dbl)  [unwired: 12 in, 1 out]
                "Downspout Flow" <- w358
                "Downspout Flow Chart" <- w358
                n173 = call "Array_Search_For_Num.vi"("N Rows of Data"=w345, "Title?"="GALLONS") -> ("number"=w359:dbl)  [unwired: 12 in, 1 out]
                "Total Flow Out" <- w359
                n174 = call "HEWH Flow Adjustment.vi"("VISA session"=w354, "Configuration"="Test Condition", "Semiphore"=w340, "GPM Target(3)"=w342, "GPM reading"=w358, "Flow rate setting In"=w369, "Error In"=w367, "Elapsed Time (sec)"=w347, "Flow Adjust Time (3s)"="Flow Adjust Time (3s)", "K(0.1)"="K(0.1)") -> ("VISA session out"=w341:refnum<visa-resource-name>, "Flow rate setting Out"=w368:dbl, "Error Out"=w348:errorcluster)  [unwired: 3 in]
                n175 = Equal To 0?(x=w353) -> (x = 0?=w350:bool)
                n176 = stacked-sequence {
                  tunnel: [w372 _ _] -> w366
                  tunnel: w359 -> [w371 _ _]
                  tunnel: [_ w373 _] -> w328
                  tunnel: [_ _ w377] -> w327
                  frame #0 {
                    n177 = local read "Gallon Limit"() -> (w370:dbl)
                    "Gallon Limit 2" <- w370
                    n178 = Greater Or Equal?(x=w371, y=w370) -> (x >= y?=w372:bool)
                  }
                  frame #1 {
                    n179 = local read "Mean Tank Min"() -> (w374:dbl)
                    "Mean Tank Min 2" <- w374
                    n180 = local read "Tank Display"() -> (w376:T5)
                    n181 = Unbundle By Name(w376) -> ("Mean"=w375:dbl)
                    n182 = Less Or Equal?(x=w375, y=w374) -> (x <= y?=w373:bool)
                  }
                  frame #2 {
                    n183 = local read "Tank Display"() -> (w380:T5)
                    n184 = local read "Min Tout"() -> (w378:dbl)
                    "Min Tout 2" <- w378
                    n185 = Unbundle By Name(w380) -> ("TOUT"=w379:dbl)
                    n186 = Less Or Equal?(x=w379, y=w378) -> (x <= y?=w377:bool)
                  }
                }
                n187 = call "HEWH Temp Adjustment.vi"("VISA session"=w341, "Semiphore"=w340, "Degrees Target(58)"=w343, "Degrees reading"=w344, "Degrees setting In"=w336, "Error In"=w348, "Elapsed Time (sec)"=w347, "Temp Adjust Time (3s)"="Flow Adjust Time (3s)", "K(0.1)"="K(0.1)") -> ("Degree setting Out"=w339:dbl, "Error Out"=w349:errorcluster)  [unwired: 4 in, 1 out]
                n188 = local read "Stop Logging"() -> (w337:bool)
                n189 = Unbundle By Name(w349) -> ("status"=w329:bool)
                n190 = Compound Arithmetic op=OR(w329, w328, w327, w366, w337) -> (w351:bool)
                n191 = Compound Arithmetic op=OR(w350, w351) -> (w352:bool)
                n192 = case shown="True" w352 {
                  tunnel: w345 -> [_ w381]
                  frame #0 {
                  }
                  frame #1 {
                    n193 = local read "FileName"() -> (w386:path)
                    n194 = Index Array(array=w381, index (row)=1) -> (element=w384:string[])  [unwired: 1 in]
                    n195 = call-poly <vilib>:"Write To Spreadsheet File.vi"("delimiter (\\t)"="," ("delimiter (\\t)"), "append to file? (new file:F)"=TRUE, "1D data"=w384, "file path (dialog if empty)"=w386) -> ()  [unwired: 4 in, 1 out]
                  }
                }
              }
              "5.Top Source Indicator" <- w305
              n196 = case shown="No Error" w309 {
                selector: w309 -> [w314 w320]
                tunnel: [w319 string[] ["Finish"] ("States")] -> w311
                tunnel: w312 -> [w319 _]
                tunnel: [w318 w320] -> w310
                tunnel: w308 -> [w317 _]
                frame #0 {
                  n197 = local read "Expansion Tank?"() -> (w316:bool)
                  n198 = local read "MW100"() -> (w313:refnum<visa-resource-name>)
                  n199 = call "HEWH Set Valves.vi"("VISA session"=w313, "Semiphore"=w317, "Expansion Tank?"=w316, "Valve Bank Setting"=ValveBankPositions."Heating", "Error In"=w314) -> ("Error Out"=w318:errorcluster)  [unwired: 9 in, 1 out]
                }
                frame #1 {
                  n200 = Unbundle By Name(w320) -> ("source"=w325:string)
                  n201 = local read "FileName"() -> (w322:path)
                  n202 = Concatenate Strings("Error: " ("string"), w325) -> (w323:string)
                  n203 = call "String_in_Reference.vi"("String"=w323) -> ("String Out"=w321:string)  [unwired: 18 in]
                  n204 = call "Log String to Spreadsheet.vi"("String"=w321, "FileName"=w322) -> ()  [unwired: 9 in, 1 out]
                  "Error 5" <- w320
                }
              }
              n205 = local write "Flowrate adj"(w301) -> ()
              n206 = local write "Temp adj"(w300) -> ()
            }
            frame #3 {
              # "Stop Serail Data"
              # "Wait till logging loop completes"
              n207 = call "YKMW100 Get Error Log.vi"("Semiphore"=w390, "error in (no error)"=w391) -> ("dup VISA session"=w393:refnum<visa-resource-name>, "Error History"=→"Error History":string[], "error out"=w394:errorcluster)  [unwired: 10 in, 1 out]
              n208 = flat-sequence {
                tunnel: w394 -> [w401]
                tunnel: w393 -> [w400]
                tunnel: w390 -> [w397]
                tunnel: [w396] -> w388
                frame #0 {
                  n209 = call "YKMW100 Get Com Log.vi"("VISA session"=w400, "Semiphore"=w397, "error in (no error)"=w401) -> ("Com History"=→"Com History":string[], "error out"=w396:errorcluster)  [unwired: 9 in, 2 out]
                  n210 = local write "Stop Logging"(TRUE ("Stop Logging")) -> ()
                }
              }
              n211 = while {
                tunnel: [TRUE ("Stop Logging")] -> w389
                tunnel: [w402] -> w387
                tunnel: w388 -> [w402]
                stop <- w405 stop-if-true
                n212 = local read "T1"() -> (w404:u32)
                n213 = Wait (ms)(milliseconds to wait=w404) -> ()  [unwired: 1 out]
                n214 = local read "St.Logging"() -> (w405:bool)
              }
              n215 = case shown="True" w389 {
                tunnel: w387 -> [_ _]
                frame #0 {
                }
                frame #1 {
                  w406 = TRUE
                  n216 = local write "StopSerial"(w406) -> ()
                  n217 = property on="StopSerial" class="Bool (strict)"("Val(Sgnl)"=w406) -> ()  [unwired: 2 in, 2 out]
                  "LoggingStopped" <- w406
                }
              }
            }
          }
          n218 = Equal?(x=w181, y="Finish") -> (x = y?=w180:bool)
        }
        n219 = while {
          tunnel: w171 -> [w419]
          shift-right: [w415] -> _
          shift-left: 0.0 -> [w412]
          i -> [w418]
          stop <- w417 stop-if-true
          n220 = local read "T4"() -> (w407:i32)
          n221 = Multiply(x=w412, y=1000.0) -> (x*y=w414:dbl)
          n222 = To Long Integer(number=w414) -> (32bit integer=w411:i32)
          n223 = Subtract(x=w407, y=w411) -> (x-y=w408:i32)
          n224 = In Range and Coerce(upper limit=w407, x=w408, lower limit=0) -> (coerced(x)=w410:i32)  [unwired: 1 out]
          n225 = event shown="[0] Timeout" {
            selector: _ -> [_]
            dyn-events: _ -> [_]
            timeout: w410 -> [_]
            tunnel: w419 -> [w459]
            tunnel: ["Stop Logging"] -> w417
            tunnel: [w424] -> w416
            event [0] Timeout {
              n226 = event-data() -> ()  [unwired: 1 in, 2 out]
              n227 = local read "Use Agilent?"() -> (w426:bool)
              n228 = local read "Chanel List"() -> (w454:string)
              n229 = flat-sequence {
                tunnel: [w461] -> w425
                tunnel: [w460] -> w424
                frame #0 {
                  n230 = local read "Label Array"() -> (w461:string[])
                  n231 = call "E-Time.vi"() -> ("Elapsed Time (sec)"=w460:dbl)  [unwired: 9 in, 2 out]
                }
              }
              n232 = local read "Serial Data In"() -> (w427:string)
              n233 = control-ref of="Tank Display"() -> (w457:refnum<vi>)
              n234 = local read "Equipment"() -> (w458:T6)
              n235 = call "Gather Test Data - Heatup Test new.vi"("Agilent Scan List"=w454, "Semiphore"=w459, "Equipment"=w458, "Tank Display Ref"=w457, "Agilent?"=w426, "Serial Data In"=w427, "Agilent Label Array"=w425) -> ("Tc Tree"=w433:dbl[], "Output Data"=w452:string[][], "POWER"=w451:T4, "PowerData"=w456:T13, "Voltage"=w423:dbl, "error out"=w430:errorcluster)  [unwired: 3 in]
              "error datalogging" <- w430
              n236 = call <vilib>:"Mean.vi"("X"=w433) -> ("mean"=→"Ave Temp":dbl)  [unwired: 1 out]
              n237 = Unbundle By Name(w456) -> ("Power"=w447:dbl)
              "Watts" <- w447
              n238 = local write "Voltage"(w423) -> ()
              n239 = Array To Cluster(array=w433) -> (cluster=w455:T14)
              n240 = Unbundle(w451) -> ("UE"=w450:bool, "LE"=w448:bool, "COMP"=w449:bool, "FANS"=w444:bool)
              n241 = Build Array(w455) -> (→"Temps":T8)
              n242 = Boolean To (0,1)(Boolean=w450) -> (0, 1=w439:i16)
              n243 = Boolean To (0,1)(Boolean=w449) -> (0, 1=w437:i16)
              n244 = Boolean To (0,1)(Boolean=w444) -> (0, 1=w443:i16)
              n245 = Boolean To (0,1)(Boolean=w448) -> (0, 1=w438:i16)
              n246 = expression code="4*x"(w439) -> (w440:i16)
              n247 = expression code="3*x"(w438) -> (w441:i16)
              n248 = expression code="2*x"(w437) -> (w442:i16)
              n249 = call "Array_Search_For_Num.vi"("N Rows of Data"=w452, "Title?"="GALLONS") -> ("number"=→"Gallons Chart" →"Gallons":dbl)  [unwired: 12 in, 1 out]
              n250 = Build Array(w447, w440, w441, w442, w443) -> (w445:dbl[])
              n251 = Array To Cluster(array=w445) -> (cluster=w446:T15)
              n252 = Build Array(w446) -> (→"Watt Chart":T9)
              n253 = local write "Test Data"(w452) -> ()
              n254 = Unbundle By Name(w430) -> ("status"=w429:bool)
              n255 = Or(x="Stop Logging", y=w429) -> (x .or. y?=w428:bool)
              n256 = case shown="True" w428 {
                selector: w428 -> [_ w468]
                tunnel: w452 -> [w463 _]
                tunnel: [w462 "" ("delimiter (\\t)")] -> _
                frame #0 {
                  w462 = "," ("delimiter (\\t)")
                  n257 = Index Array(array=w463, index (row)=1) -> (element=w465:string[])  [unwired: 1 in]
                  n258 = local read "FileName"() -> (w467:path)
                  n259 = call-poly <vilib>:"Write To Spreadsheet File.vi"("delimiter (\\t)"=w462, "append to file? (new file:F)"=TRUE, "1D data"=w465, "file path (dialog if empty)"=w467) -> ()  [unwired: 4 in, 1 out]
                }
                frame #1 {
                  n260 = local write "Stop Logging"(w468) -> ()
                  n261 = property on="Stop Logging" class="Bool (strict)"("Val(Sgnl)"=w468) -> ()  [unwired: 2 in, 2 out]
                  "St.Logging" <- w468
                }
              }
            }
          }
          n262 = flat-sequence {
            tunnel: w416 -> [w421]
            tunnel: [w420] -> w415
            frame #0 {
              n263 = call "E-Time.vi"() -> ("Elapsed Time (sec)"=w422:dbl)  [unwired: 9 in, 2 out]
              n264 = Subtract(x=w422, y=w421) -> (x-y=w420:dbl)
            }
          }
          "Number of Records" <- w418
        }
      }
      frame #2 {
        w470 = TRUE ("Stop Logging")
        n265 = local write "Stop Logging"(w470) -> ()
        n266 = property on="Stop Logging" class="Bool (strict)"("Val(Sgnl)"=w470) -> ()  [unwired: 2 in, 2 out]
        n267 = case shown="Error" w472 {
          selector: w472 -> [w477 w484]
          tunnel: [w478 string[] ["Finish"] ("States")] -> w474
          tunnel: w475 -> [w478 _]
          tunnel: [w477 w484] -> w476
          frame #0 {
          }
          frame #1 {
            n268 = Unbundle By Name(w484) -> ("source"=w479:string)
            n269 = local read "FileName"() -> (w482:path)
            n270 = Concatenate Strings("Error: " ("string"), w479) -> (w481:string)
            n271 = call "String_in_Reference.vi"("String"=w481) -> ("String Out"=w483:string)  [unwired: 18 in]
            n272 = call "Log String to Spreadsheet.vi"("String"=w483, "FileName"=w482) -> ()  [unwired: 9 in, 1 out]
          }
        }
      }
    }
    n273 = Equal?(x=w19, y="Finish") -> (x = y?=w27:bool)
  }
  "Error Out" <- w6
  n274 = flat-sequence {
    tunnel: w1 -> [_]
    frame #0 {
      w486 = TRUE ("stop")
      n275 = call "String_in_Reference.vi"("String"="Stopping Test") -> ()  [unwired: 18 in, 1 out]
      n276 = local write "Stop"(w486) -> ()
      n277 = property on="Stop" class="Bool (strict)"("Val(Sgnl)"=w486) -> ()  [unwired: 2 in, 2 out]
    }
  }
  n278 = while {
    stop <- w489 stop-if-true
    n279 = local read "T2"() -> (w488:u32)
    n280 = event shown="[1] \"Stop\": Value Change" {
      selector: _ -> [_ _ _]
      dyn-events: _ -> [_ _ _]
      timeout: w488 -> [_ _ _]
      tunnel: [FALSE ("stop? (T)") w493 FALSE ("stop? (T)")] -> w489
      event #0 {
        n281 = event-data() -> ()  [unwired: 1 in, 2 out]
        n282 = call "E-Time.vi"() -> ("Elapsed Time (sec)"=→"Elapsed Time":dbl)  [unwired: 9 in, 2 out]
        n283 = call "String_in_Reference.vi"() -> ("String Out"=→"MINI-HEATUP TEST STATUS":string)  [unwired: 19 in]
      }
      event #1 {
        n284 = event-data() -> ()  [unwired: 1 in, 5 out]
        n285 = case shown="True" "Stop" {
          tunnel: [FALSE ("stop? (T)") w496] -> w493
          frame #0 {
          }
          frame #1 {
            n286 = stacked-sequence {
              tunnel: [_ _ _ _ TRUE ("stop? (T)")] -> w496
              frame #0 {
                # "Open outlet valve."
                n287 = local read "Semiphore"() -> (w500:T3)
                n288 = local read "MW100"() -> (w499:refnum<visa-resource-name>)
                n289 = call "HEWH Set Valves.vi"("VISA session"=w499, "Semiphore"=w500, "Expansion Tank?"="Expansion Tank?", "Valve Bank Setting"=ValveBankPositions."Resting") -> ()  [unwired: 10 in, 2 out]
              }
              frame #1 {
                n290 = local read "Local?"() -> (w501:bool)
                n291 = case shown="True" w501 {
                  tunnel: w501 -> [_ w502]
                  frame #0 {
                  }
                  frame #1 {
                    n292 = local read "Equipment"() -> (w505:T6)
                    n293 = local read "Semiphore"() -> (w504:T3)
                    n294 = call "HEWH CloseEquipmet.vi"("Semiphore"=w504, "Equipment"=w505) -> ("Error Out"=w503:errorcluster)  [unwired: 9 in]
                    n295 = call "Semiphore-Destroy-Local.vi"("Semiphore"=w504, "Local?"=w502, "error in (no error)"=w503) -> ()  [unwired: 16 in, 1 out]
                  }
                }
              }
              frame #2 {
                n296 = local read "FileName"() -> (w506:path)
                n297 = local read "Init Complete"() -> (w508:bool)
                n298 = call <vilib>:"Check if File or Folder Exists.vi"("path"=w506) -> ("file or folder exists?"=w509:bool)  [unwired: 8 in, 2 out]
                n299 = And(x=w509, y=w508) -> (x .and. y?=w507:bool)
                n300 = case shown="True" w507 {
                  tunnel: w506 -> [_ w514]
                  frame #0 {
                  }
                  frame #1 {
                    n301 = Strip Path(path=w514) -> (name=w513:string)  [unwired: 1 out]
                    n302 = Search and Replace String(input string=w513, search string=".tmp", replace string=".csv" ("search string")) -> (result string=w511:string, error out=w517:errorcluster)  [unwired: 5 in, 2 out]
                    n303 = Build Path(base path="Save File Directory", name or relative path=w511) -> (appended path=w510:path)
                    n304 = Move(source path=w514, error in=w517, 10:w510) -> ()  [unwired: 2 in, 3 out]
                  }
                }
              }
              frame #3 {
                n305 = local write "Stop"(FALSE ("stop")) -> ()
                n306 = local write "MINI-HEATUP TEST STATUS"("Complete OK" ("STATUS")) -> ()
              }
              frame #4 {
                w526 = ","
                n307 = local read "Computer Name"() -> (w525:string)
                n308 = local read "LAN IP Address"() -> (w521:string)
                n309 = local read "Ver."() -> (w524:string)
                n310 = property class="App"() -> ("App.Name"=w522:string)  [unwired: 2 in, 2 out]
                n311 = Concatenate Strings(w521, w526, w525, w526, w522, w526, w524, w526, "Stopped." ("string")) -> (w520:string)
                n312 = call "Save Time to File.vi"("String"=w520) -> ()  [unwired: 13 in, 2 out]
              }
            }
          }
        }
      }
      event #2 {
        n313 = event-data() -> ()  [unwired: 1 in, 1 out]
        n314 = One Button Dialog(message="\n1.\tAfter unit has been stable for 30+/-5 minutes, Open valve, and draw 10.75 +/- .25 gallons of water at a rate of 3+/-.25 gpm.\n2.\tIf lower heat source energizes (Hybrid Mode/eHeat Mode = FAN ON follow by Compressor, Standard Electric Mode = Lower Element ON) before 10.75 gallons, then continue drawing water until Upper element engages as shown in step 5 (skip to step 5).\n3.\tIf lower heat source does not energize during 10.75 gallon draw, then wait a maximum of 10 minutes to see if lower heat source will energize.  If it does, then allow the water heater to recover to set point.\n4.\tAllow unit to sit 5 to 10 minutes in stabilized conditions, then:\n5.\tOpen valve and draw water at 3+/-.25 gpm until the Upper Element energizes.  Water draw must stop within 5 seconds after Upper Element energizes.  NOTE: when running the unit in e-Heat mode, (no upper element) draw 40+/-0.25 gallons of water.\n6.\tIn Hybrid Mode: when the Upper Element stops and switches to Lower Element, switch the unit to eHeat Mode.  This will switch the lower heating source to Compressor.\n7.\tAllow water heater to stabilize this second time. (Recover water temperature back to set point).\n8.\tAllow unit to sit a minimum of 30 minutes in stabilized conditions, then;\n9.\tStop Data Logger and HyperTerminal session. \n10.\tCapture all data into format shown in attached spreadsheet.\n\n\n") -> (true=w531:bool)  [unwired: 1 in]
        n315 = Not(x=w531) -> (.not. x?=w530:bool)
        n316 = local write "Help"(w530) -> ()
      }
    }
  }
